vi "save peaks.vi"(0 "save":bool, 1 "base path":path=path "C:/Documents and Settings/weitzlab/Desktop", 2 "peaks data":T1, 3 "Acq Rate [Hz]":dbl=100000.0 min=1.0 max=200000.0 step=1.0 format="%#_6p", 5 "column titles":string[](array[string])=["Max 1 [volts]", "Max 2 [volts]", "Max 3 [volts]", "Max 4 [volts]", "<Height 1> [volts]", "<Height 2> [volts]", "<Height 3> [volts]", "<Height 4> [volts]", "Time inside [ms]", "Time outside [ms]", "Sa/Sb or MaxSa"], 7 "filename":string="peaks_", 12 "shifts in":cluster{"save":bool, dbl, "appended path":path}) -> (4 "save!":bool, 6 "number of files":i32, 8 "path to file":path, 14 "shifts out":cluster{"save":bool, dbl, "appended path":path})   [LabVIEW 2009]
uses:
  <vilib>/Utility/file.llb/Write To Spreadsheet File (string).vi
panel:
  out "?":string
  out "same file as before":bool
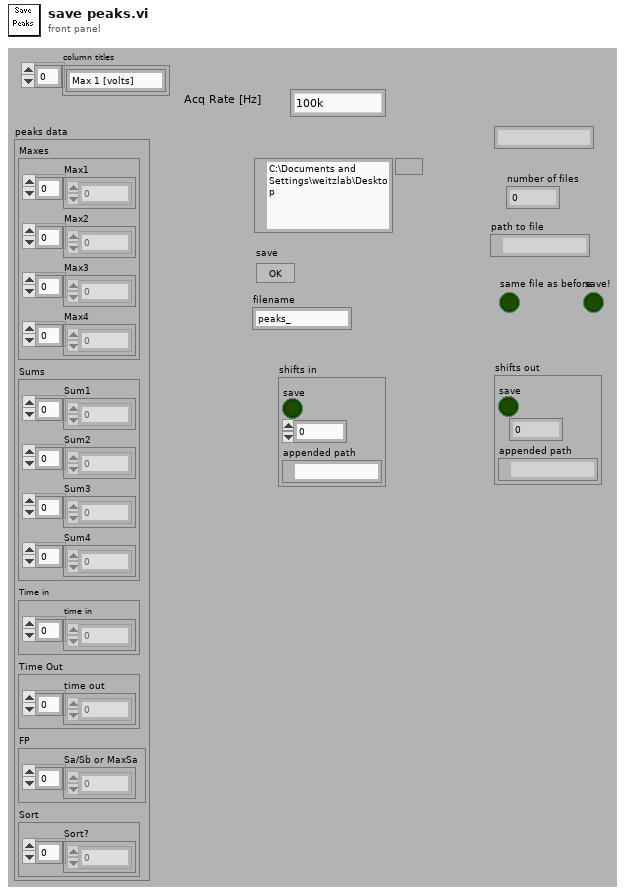
[diagram p1: front panel]
types:
  T1 = cluster{"Maxes":cluster{"Max1":dbl[], "Max2":dbl[], "Max3":dbl[], "Max4":dbl[]}, "Sums":cluster{"Sum1":dbl[], "Sum2":dbl[], "Sum3":dbl[], "Sum4":dbl[]}, "Time in":cluster{"time in":dbl[]}, "Time Out":cluster{"time out":dbl[]}, "FP":cluster{"Sa/Sb or MaxSa":dbl[]}, "Sort":cluster{"Sort?":dbl[]}}
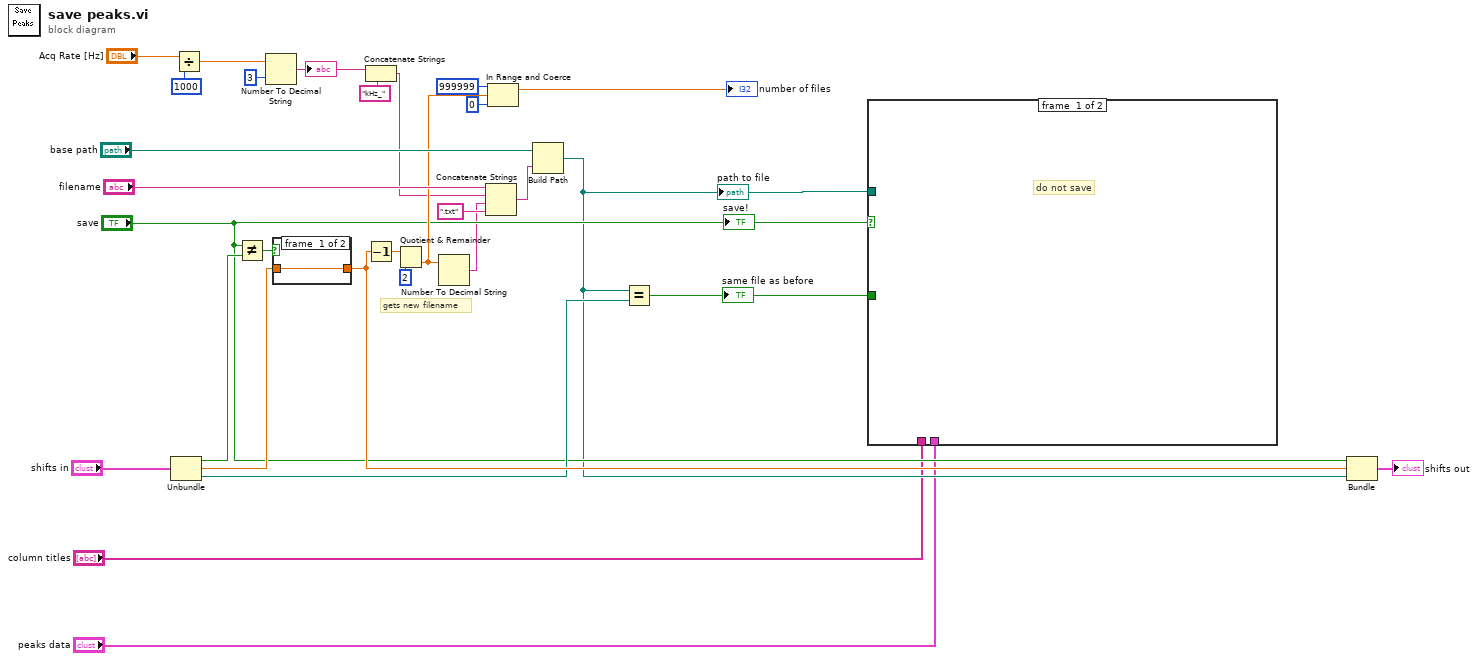
[diagram p0: block diagram]
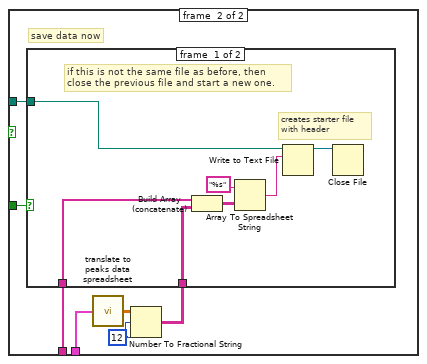
[diagram p2: hidden frame]
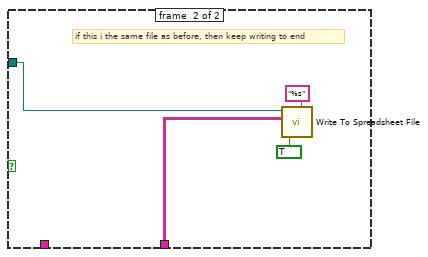
[diagram p3: hidden frame]
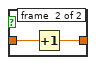
[diagram p4: hidden frame]
diagram:
  # "gets new filename"
  n1 = Unbundle("shifts in") -> ("save"=w24:bool, w25:dbl, "appended path"=w17:path)
  n2 = Divide(x="Acq Rate [Hz]", y=1000) -> (x/y=w8:dbl)
  n3 = Not Equal?(x="save", y=w24) -> (x != y?=w29:bool)
  n4 = Number To Decimal String(number=w8, width (-)=i16 3) -> (decimal integer string=w6:string)
  "?" <- w6
  n5 = case shown="False" w29 {
    tunnel: [w31 w33] -> w26
    tunnel: w25 -> [w31 w32]
    frame #0 {
    }
    frame #1 {
      n6 = Increment(x=w32) -> (x+1=w33:dbl)
    }
  }
  n7 = Concatenate Strings(w6, "kHz_" ("string")) -> (w4:string)
  n8 = Decrement(x=w26) -> (x-1=w27:dbl)
  n9 = Quotient & Remainder(x=w27, y=2) -> (floor(x/y)=w21:dbl)  [unwired: 1 out]
  n10 = Number To Decimal String(number=w21) -> (decimal integer string=w9:string)  [unwired: 1 in]
  n11 = Concatenate Strings("filename", w4, w9, ".txt" ("string")) -> (w22:string)
  n12 = In Range and Coerce(upper limit=999999, x=w21, lower limit=0) -> (coerced(x)=→"number of files":dbl)  [unwired: 1 out]
  n13 = Build Path(base path="base path", name or relative path=w22) -> (appended path=w13:path)
  "path to file" <- w13
  n14 = Equal?(x=w13, y=w17) -> (x = y?=w15:bool)
  "same file as before" <- w15
  n15 = case shown="True" "save" {
    tunnel: w15 -> [_ w40]
    tunnel: w13 -> [_ w39]
    tunnel: "column titles" -> [_ w38]
    tunnel: "peaks data" -> [_ w35]
    frame #0 {
      # "do not save"
    }
    frame #1 {
      w37 = i16 12 ("precision (6)")
      # "save data now"
      n16 = call "translate to peaks data spreadsheet.vi"("peaks data"=w35) -> ("peaks data"=w36:dbl[][])  [unwired: 14 in]
      n17 = Number To Fractional String(number=w36, width (-)=w37, precision (6)=w37) -> (F-format string=w34:string[][])  [unwired: 1 in]
      n18 = case shown="True" w40 {
        tunnel: w39 -> [w47 w49]
        tunnel: w38 -> [w45 _]
        tunnel: w34 -> [w41 w48]
        frame #0 {
          # "creates starter file\nwith header"
          # "if this is not the same file as before, then close the previous file and start a new one."
          n19 = Build Array (concatenate)(w45, w41) -> (w46:string[][])
          n20 = Array To Spreadsheet String(array=w46, 3:"%s" ("format string")) -> (spreadsheet string=w44:string)  [unwired: 1 in]
          n21 = Write to Text File(file (use dialog)=w47, text=w44) -> (refnum out=w42:refnum<file>)  [unwired: 2 in, 2 out]
          n22 = Close File(refnum=w42) -> ()  [unwired: 1 in, 2 out]
        }
        frame #1 {
          # "if this i the same file as before, then keep writing to end"
          n23 = call-poly <vilib>:"Write To Spreadsheet File.vi"("format (%s)"="%s", "append to file? (new file:F)"=TRUE, "2D data"=w48, "file path (dialog if empty)"=w49) -> ()  [unwired: 4 in, 1 out]
        }
      }
    }
  }
  n24 = Bundle("save"="save", w26, "appended path"=w13) -> (→"shifts out":cluster{"save":bool, dbl, "appended path":path})  [unwired: 1 in]
  "save!" <- "save"
